vi "softmax_demo.vi"() -> ()   [LabVIEW 2014]
uses:
  <vilib>/Analysis/Matrix/Datatypes/RealMatrix.ctl
  <vilib>/Analysis/baseanly.llb/Real A x B.vi
  <vilib>/Analysis/Matrix/Numeric/Add/Add - RM,RM.vi
  <vilib>/Analysis/NI_AALBase.lvlib
  <vilib>/Analysis/Matrix/NI_Matrix.lvlib
panel:
  out "y":T1
  out "max index":i32
  out "softmax":T1
  out "sum(e^y)":dbl
  out "e^y":T1
  out "b":T1
  in  "seed_ix":i32
  out "max value":dbl
  out "Wxh * h":T1
  out "h":T1
  out "Wxh":T1
  in  "nCols":i32
  in  "nRows":i32
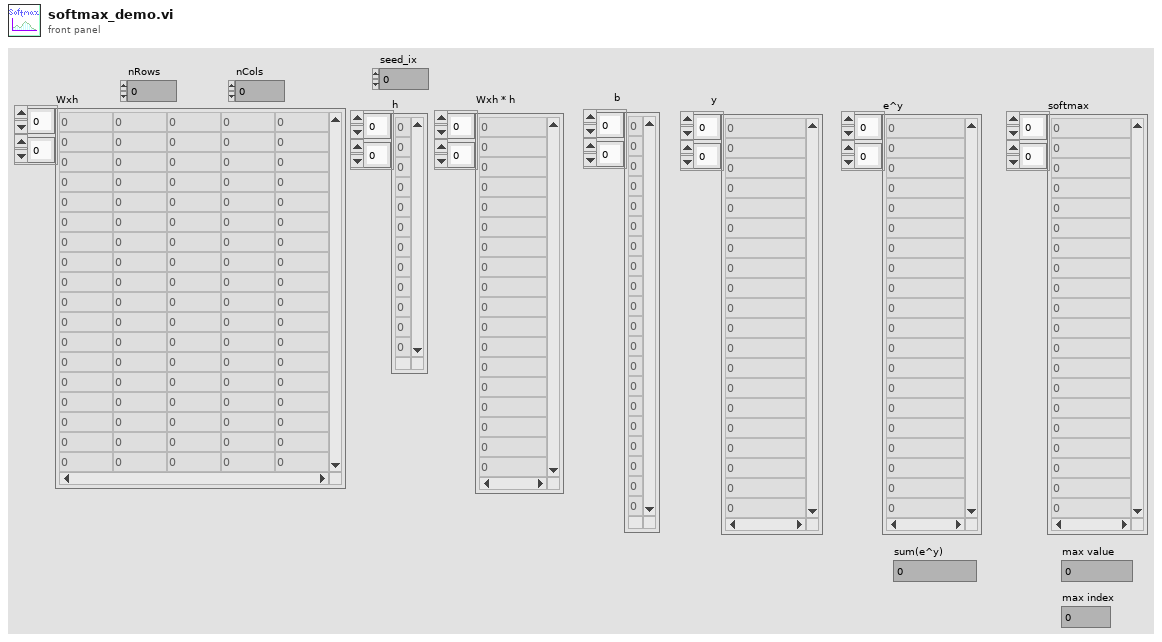
[diagram p1: front panel]
types:
  T1 = typedef "NI_Matrix.lvlib/RealMatrix.ctl" = dbl[][]
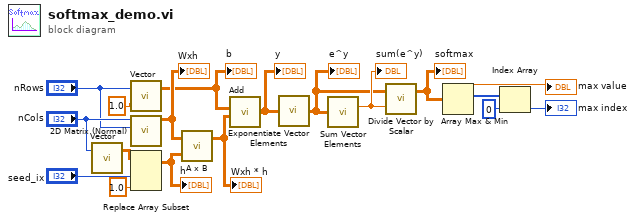
[diagram p0: block diagram]
diagram:
  n1 = call "Vector.vi"("length"="nCols") -> ("Real Matrix (Column Vector)"=w11:T1)  [unwired: 18 in]
  n2 = call "Vector.vi"("length"="nRows", "element (0)"=1.0 ("element")) -> ("Real Matrix (Column Vector)"=w2:T1)  [unwired: 17 in]
  "b" <- w2
  n3 = call "2D Matrix (Normal).vi"("nRows"="nRows", "nCols"="nCols") -> ("Normal Matrix"=w17:T1)  [unwired: 9 in]
  "Wxh" <- w17
  n4 = Replace Array Subset(array=w11, new element=1.0 ("new element/submatrix"), index (row)="seed_ix") -> (w9:T1)  [unwired: 1 in]
  "h" <- w9
  n5 = call-poly <vilib>:"A x B.vi"("B"=w9, "A"=w17) -> ("A x B"=w1:T1)  [unwired: 1 out]
  "Wxh * h" <- w1
  n6 = call-poly <vilib>:"Add.vi"("Real Matrix B"=w1, "Real Matrix A"=w2) -> ("A + B"=w13:T1)
  "y" <- w13
  n7 = call "Exponentiate Vector Elements.vi"("X"=w13) -> ("exp(X)"=w6:T1)
  "e^y" <- w6
  n8 = call "Sum Vector Elements.vi"("A x B"=w6) -> ("Numeric"=w7:dbl)
  "sum(e^y)" <- w7
  n9 = call "Divide Vector by Scalar.vi"("Vector"=w6, "x"=w7) -> ("Scaled Vector"=w8:T1)  [unwired: 17 in]
  "softmax" <- w8
  n10 = Array Max & Min(array=w8) -> (max value=→"max value":dbl, max index (indices)=w5:i32[])  [unwired: 2 out]
  n11 = Index Array(array=w5, index=0) -> (element=→"max index":i32)
